vi "Main.vi"() -> ()   [LabVIEW 2016]
doc: "DACELL DN-10W load cell indicator \nmodbus communication program \n*function mode: Decision mode\n\nget display value\nget relay set value\nget physical unit\nset relay set value\n\nloop time 500 ms"
uses:
  Ctl/ctl_state.ctl
  <vilib>/NI/Modbus Library/API/Master/Modbus Master.lvclass
  <vilib>/Utility/error.llb/DialogType.ctl
panel:
  out "State":T1
  out "Error Out":errorcluster caption="에러 출력"
  in  "Error In":errorcluster caption="에러 입력"
  out "Run?":bool
  out "Connected?":bool
  in  "end":bool
  in  "zero":bool
  in  "update":bool
  in  "read":bool
  in  "disconnect":bool
  in  "connect":bool
  in  "Set velue":dbl=18.9 format="%#.1g"
  out "Unit":string="kgf"
  out "High limit":dbl
  out "Low limit":dbl
  out "relay3":bool
  out "relay2":bool
  out "relay1":bool
  out "Present value":dbl
  in  "baud rate":u32=9600
  in  "unit ID":u8=2
  in  "VISA resource name":refnum<visa-resource-name>
  # "DACELL DN-10W \nMODBUS Communication Program"
  # "DACELL DN-10W indicator MODBUS-RTU by Kyuman Kim"
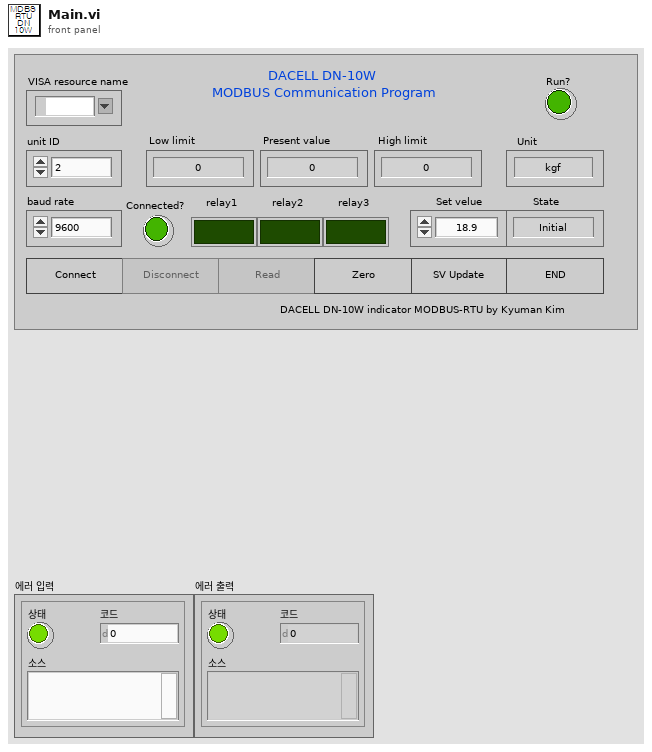
[diagram p1: front panel]
types:
  T1 = typedef "ctl_state.ctl" = enum16{"Initial", "Wait", "Connect", "Disconnect", "Read", "Update", "Zero", "End"}
  T2 = enum8{"Enabled", "Disabled", "Disabled and Grayed Out"}
  T3 = typedef "DialogType.ctl" = u16
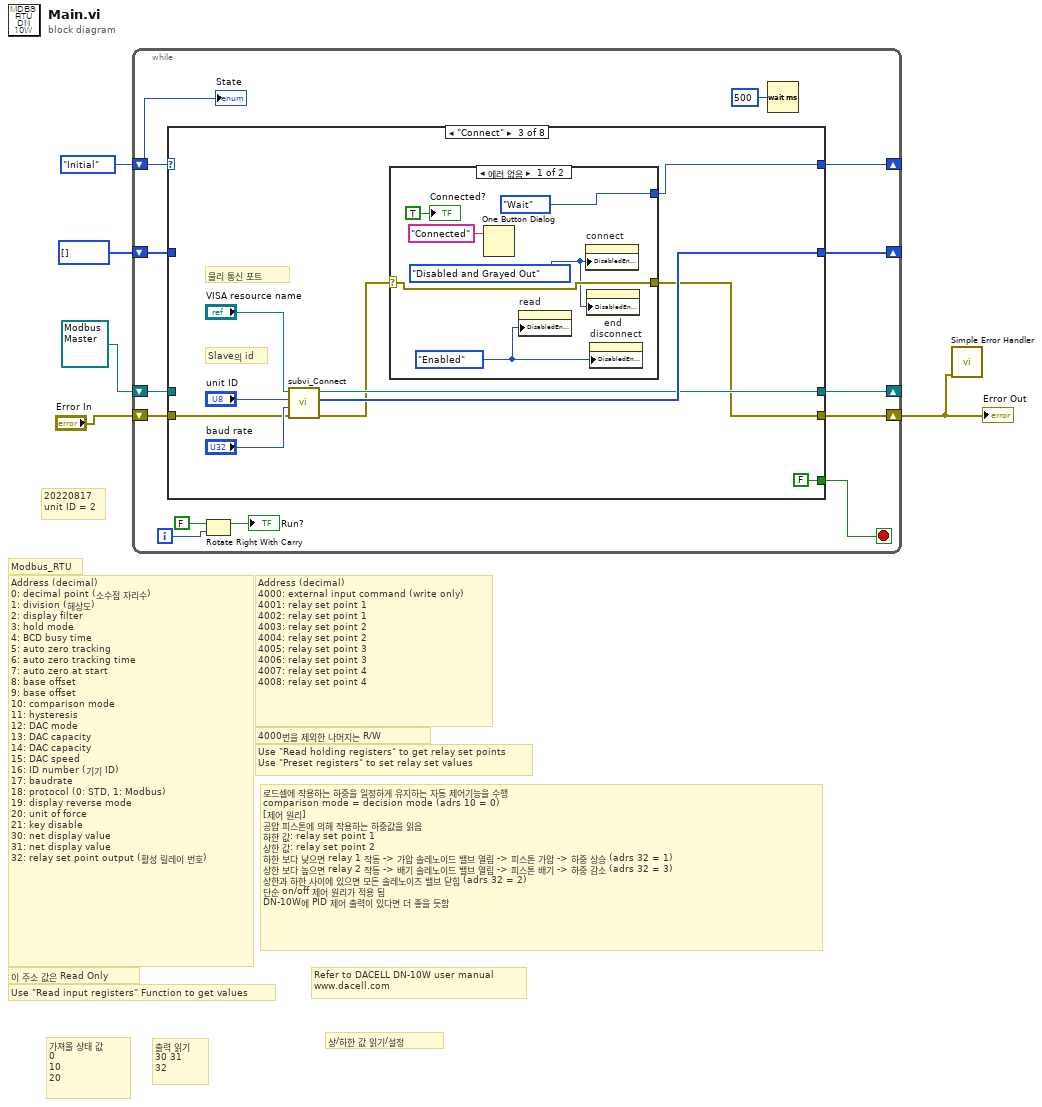
[diagram p0: block diagram]
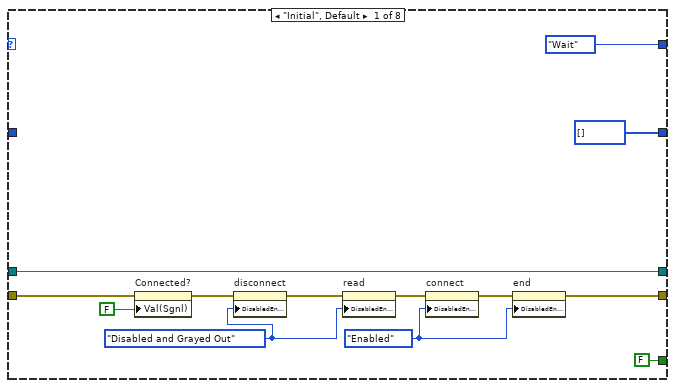
[diagram p2: hidden frame]
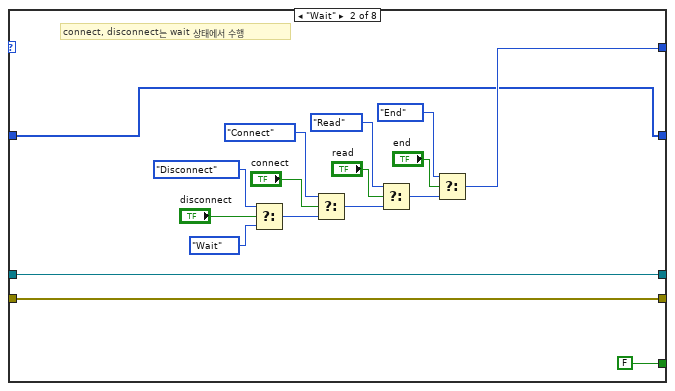
[diagram p3: hidden frame]
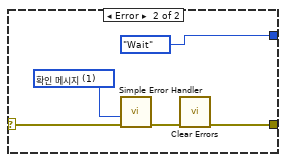
[diagram p4: hidden frame]
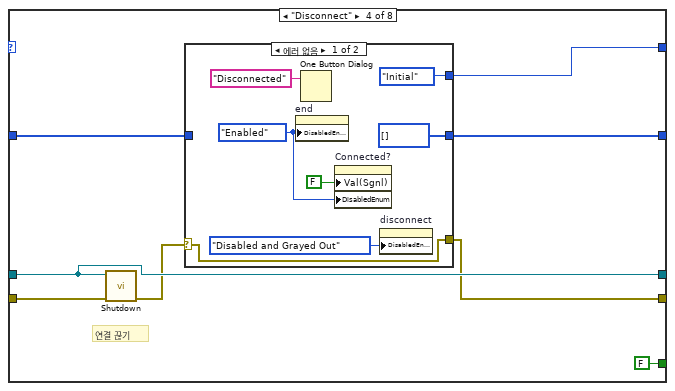
[diagram p5: hidden frame]
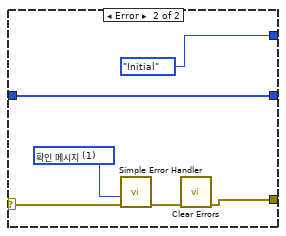
[diagram p6: hidden frame]
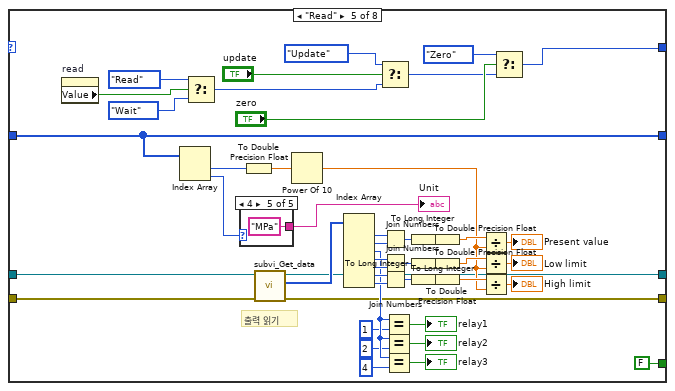
[diagram p7: hidden frame]
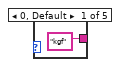
[diagram p8: hidden frame]
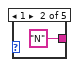
[diagram p9: hidden frame]
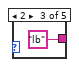
[diagram p10: hidden frame]
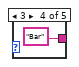
[diagram p11: hidden frame]
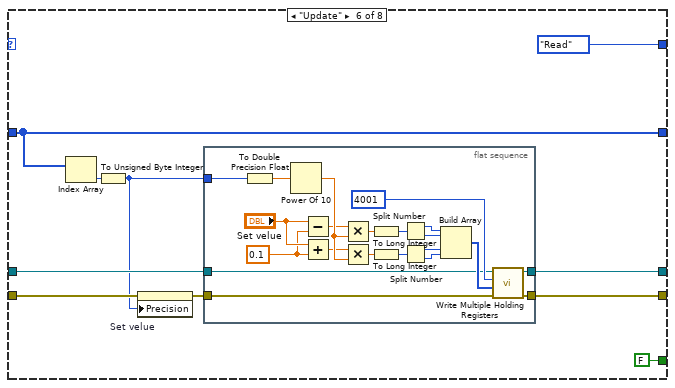
[diagram p12: hidden frame]
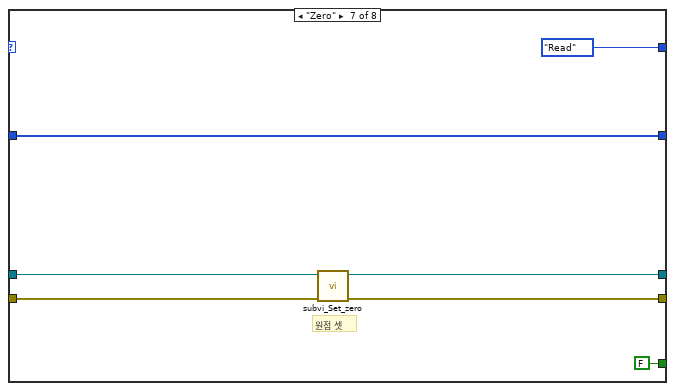
[diagram p13: hidden frame]
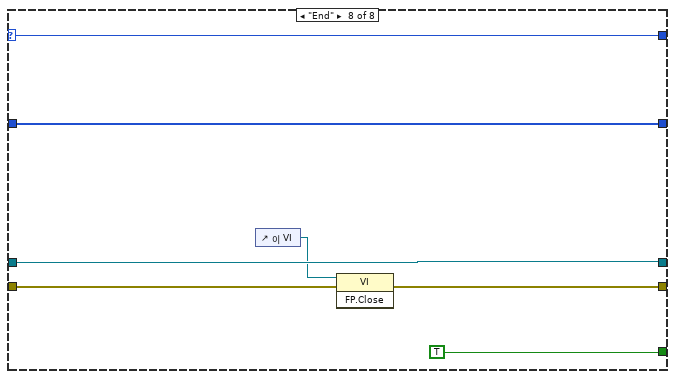
[diagram p14: hidden frame]
diagram:
  # "20220817\nunit ID = 2"
  # "상/하한 값 읽기/설정"
  # "출력 읽기\n30 31\n32"
  # "가져올 상태 값\n0\n10\n20"
  # "로드셀에 작용하는 하중을 일정하게 유지하는 자동 제어기능을 수행\ncomparison mode = decision mode (adrs 10 = 0)\n[제어 원리]\n공압 피스톤에 의해 작용하는 하중값을 읽음\n하한 값: relay set point 1\n상한 값: relay set point 2\n하한 보다 낮으면 relay 1 작동 -> 가압 솔레노이드 밸브 열림 -> 피스톤 가압 -> 하중 상승 (adrs 32 = 1)\n상한 보다 높으면 relay 2 작동 -> 배기 솔레노이드 밸브 열림 -> 피스톤 배기 -> 하중 감소 (adrs 32 = 3)\n상한과 하한 사이에 있으면 모든 솔레노이즈 밸브 닫힘 (adrs 32 = 2)\n단순 on/off 제어 원리가 적용 됨\nDN-10W에 PID 제어 출력이 있다면 더 좋을 듯함"
  # "4000번을 제외한 나머지는 R/W"
  # "이 주소 값은 Read Only"
  # "Modbus_RTU"
  # "Refer to DACELL DN-10W user manual\nwww.dacell.com"
  # "Use \"Read holding registers\" to get relay set points\nUse \"Preset registers\" to set relay set values"
  # "Use \"Read input registers\" Function to get values"
  # "Address (decimal)\n4000: external input command (write only)\n4001: relay set point 1 \n4002: relay set point 1\n4003: relay set point 2\n4004: relay set point 2\n4005: relay set point 3\n4006: relay set point 3\n4007: relay set point 4\n4008: relay set point 4"
  # "Address (decimal)\n0: decimal point (소수점 자리수)\n1: division (해상도)\n2: display filter\n3: hold mode\n4: BCD busy time\n5: auto zero tracking\n6: auto zero tracking time\n7: auto zero at start\n8: base offset\n9: base offset\n10: comparison mode \n11: hysteresis\n12: DAC mode\n13: DAC capacity\n14: DAC capacity\n15: DAC speed\n16: ID number (기기 ID)\n17: baudrate \n18: protocol (0: STD, 1: Modbus)\n19: display reverse mode\n20: unit of force\n21: key disable\n30: net display value \n31: net display value\n32: relay set point output (활성 릴레이 번호)"
  n1 = while {
    shift-right: [w16] -> w1
    shift-left: "Error In" -> [w17]
    shift-right: [w15] -> _
    shift-left: u16[] [] ("register values") -> [w12]
    shift-right: [w14] -> _
    shift-left: refnum<class "Modbus Master.lvclass"> refnum ("Modbus Master 출력") -> [w13]
    shift-right: [w11] -> _
    shift-left: ctl_state."Initial" ("열거형") -> [w18]
    i -> [w8]
    stop <- w10 stop-if-true
    n2 = case shown="\"Connect\"" w18 {
      selector: w18 -> [_ _ _ _ _ _ _ w184]
      tunnel: w17 -> [w23 w47 w55 w77 w91 w148 w178 w186]
      tunnel: [w19 w47 w49 w70 w106 w143 w174 w185] -> w16
      tunnel: [u16[] [] ("register values") w33 w54 w73 w103 w149 w177 w187] -> w15
      tunnel: [w31 w48 w53 w76 w104 w150 w179 w182] -> w14
      tunnel: w13 -> [w31 w48 _ w76 w105 w151 w180 w182]
      tunnel: w12 -> [_ w33 _ w74 w103 w149 w177 w187]
      tunnel: [ctl_state."Wait" ("열거형") w34 w52 w75 w94 ctl_state."Read" ("열거형") ctl_state."Read" ("열거형") w184] -> w11
      tunnel: [FALSE FALSE FALSE FALSE FALSE FALSE FALSE TRUE] -> w10
      frame "Initial", Default {
        w25 = T2."Enabled" ("비활성화")
        w26 = T2."Disabled and Grayed Out" ("비활성화")
        n3 = property on="Connected?" class="Bool (엄격한)"(error in=w23, "Val(Sgnl)"=FALSE ("값(신호)")) -> (error out=w30:errorcluster)  [unwired: 1 in, 1 out]
        n4 = property on="disconnect" class="Bool"(error in=w30, "DisabledEnum"=w26) -> (error out=w22:errorcluster)  [unwired: 1 in, 1 out]
        n5 = property on="read" class="Bool (엄격한)"(error in=w22, "DisabledEnum"=w26) -> (error out=w21:errorcluster)  [unwired: 1 in, 1 out]
        n6 = property on="connect" class="Bool"(error in=w21, "DisabledEnum"=w25) -> (error out=w20:errorcluster)  [unwired: 1 in, 1 out]
        n7 = property on="end" class="Bool"(error in=w20, "DisabledEnum"=w25) -> (error out=w19:errorcluster)  [unwired: 1 in, 1 out]
      }
      frame "Wait" {
        # "connect, disconnect는 wait 상태에서 수행"
        n8 = Select(t=ctl_state."Disconnect" ("열거형"), s="disconnect", f=ctl_state."Wait" ("열거형")) -> (s? t:f=w44:T1)
        n9 = Select(t=ctl_state."Connect" ("열거형"), s="connect", f=w44) -> (s? t:f=w40:T1)
        n10 = Select(t=ctl_state."Read" ("열거형"), s="read", f=w40) -> (s? t:f=w36:T1)
        n11 = Select(t=ctl_state."End" ("열거형"), s="end", f=w36) -> (s? t:f=w34:T1)
      }
      frame "Connect" {
        # "물리 통신 포트"
        # "Slave의 id"
        n12 = call "subvi_Connect.vi"("에러"=w55, "baud rate"="baud rate", "unit ID"="unit ID", "VISA 참조 번호 입력"="VISA resource name") -> ("에러 출력"=w50:errorcluster, "register values"=w54:u16[], "Modbus Master 출력"=w53:refnum<class "Modbus Master.lvclass">)  [unwired: 5 in]
        n13 = case shown="에러 없음" w50 {
          selector: w50 -> [w64 w68]
          tunnel: [ctl_state."Wait" ("열거형") ctl_state."Wait" ("열거형")] -> w52
          tunnel: [w64 w65] -> w49
          frame No Error {
            w59 = T2."Enabled" ("비활성화")
            w60 = T2."Disabled and Grayed Out" ("비활성화")
            n14 = One Button Dialog(message="Connected" ("메시지")) -> ()  [unwired: 1 in, 1 out]
            n15 = property on="read" class="Bool (엄격한)"("DisabledEnum"=w59) -> ()  [unwired: 2 in, 2 out]
            n16 = property on="connect" class="Bool"("DisabledEnum"=w60) -> ()  [unwired: 2 in, 2 out]
            n17 = property on="end" class="Bool"("DisabledEnum"=w60) -> ()  [unwired: 2 in, 2 out]
            n18 = property on="disconnect" class="Bool"("DisabledEnum"=w59) -> ()  [unwired: 2 in, 2 out]
            "Connected?" <- TRUE ("Connected?")
          }
          frame Error {
            w67 = T3 1 items=["대화 상자 없음", "확인 메시지", "메시지 지속 또는 정지", "확인 메시지 + 경고", "지속/정지 + 경고"] ("type of dialog (OK msg:1)")
            n19 = call <vilib>:"Simple Error Handler.vi"("type of dialog (OK msg:1)"=w67, "error in (no error)"=w68) -> ("error out"=w66:errorcluster)  [unwired: 3 in, 4 out]
            n20 = call <vilib>:"Clear Errors.vi"("error in (no error)"=w66) -> ("error out"=w65:errorcluster)  [unwired: 5 in, 1 out]
          }
        }
      }
      frame "Disconnect" {
        # "연결 끊기"
        n21 = call-dynamic "Shutdown.vi"("error in"=w77, "Modbus master in"=w76) -> ("error out"=w71:errorcluster)  [unwired: 9 in]
        n22 = case shown="에러 없음" w71 {
          selector: w71 -> [w78 w89]
          tunnel: [ctl_state."Initial" ("열거형") ctl_state."Initial" ("열거형")] -> w75
          tunnel: w74 -> [_ w87]
          tunnel: [u16[] [] ("register values") w87] -> w73
          tunnel: [w78 w85] -> w70
          frame No Error {
            w80 = T2."Enabled" ("비활성화")
            n23 = property on="end" class="Bool"("DisabledEnum"=w80) -> ()  [unwired: 2 in, 2 out]
            n24 = One Button Dialog(message="Disconnected" ("메시지")) -> ()  [unwired: 1 in, 1 out]
            n25 = property on="Connected?" class="Bool (엄격한)"("Val(Sgnl)"=FALSE ("값(신호)"), "DisabledEnum"=w80) -> ()  [unwired: 2 in, 2 out]
            n26 = property on="disconnect" class="Bool"("DisabledEnum"=T2."Disabled and Grayed Out" ("비활성화")) -> ()  [unwired: 2 in, 2 out]
          }
          frame Error {
            w88 = T3 1 items=["대화 상자 없음", "확인 메시지", "메시지 지속 또는 정지", "확인 메시지 + 경고", "지속/정지 + 경고"] ("type of dialog (OK msg:1)")
            n27 = call <vilib>:"Simple Error Handler.vi"("type of dialog (OK msg:1)"=w88, "error in (no error)"=w89) -> ("error out"=w86:errorcluster)  [unwired: 3 in, 4 out]
            n28 = call <vilib>:"Clear Errors.vi"("error in (no error)"=w86) -> ("error out"=w85:errorcluster)  [unwired: 5 in, 1 out]
          }
        }
      }
      frame "Read" {
        # "출력 읽기"
        n29 = property on="read" class="Bool (엄격한)"() -> ("Value"=w93:bool)  [unwired: 2 in, 2 out]
        n30 = Index Array(array=w103) -> (element #1=w137:u16, element #2=w125:u16)  [unwired: 2 in]
        n31 = Select(t=ctl_state."Read" ("열거형"), s=w93, f=ctl_state."Wait" ("열거형")) -> (s? t:f=w98:T1)
        n32 = case shown="4" w125 {
          tunnel: ["kgf" "N" "lb" "Bar" "MPa"] -> w124
          frame 0, Default {
          }
          frame 1 {
          }
          frame 2 {
          }
          frame 3 {
          }
          frame 4 {
          }
        }
        "Unit" <- w124
        n33 = To Double Precision Float(number=w137) -> (double precision float=w123:dbl)
        n34 = call "subvi_Get_data.vi"("에러 입력(에러 없음)"=w91, "Modbus Master 입력"=w105) -> ("에러 출력"=w106:errorcluster, "register values"=w107:u16[], "Modbus Master 출력"=w104:refnum<class "Modbus Master.lvclass">)  [unwired: 7 in]
        n35 = Power Of 10(x=w123) -> (10^x=w133:dbl)
        n36 = Index Array(array=w107) -> (element #1=w109:u16, element #2=w108:u16, element #3=w115:u16, element #4=w126:u16, element #5=w127:u16, element #6=w128:u16, element #7=w129:u16)  [unwired: 7 in]
        n37 = Select(t=ctl_state."Update" ("열거형"), s="update", f=w98) -> (s? t:f=w95:T1)
        n38 = Join Numbers(hi=w109, lo=w108) -> ((hi.lo)=w110:u32)
        n39 = Join Numbers(hi=w126, lo=w127) -> ((hi.lo)=w119:u32)
        n40 = Join Numbers(hi=w128, lo=w129) -> ((hi.lo)=w120:u32)
        n41 = Equal?(x=w115, y=u16 1) -> (x = y?=→"relay1":bool)
        n42 = Equal?(x=w115, y=u16 2) -> (x = y?=→"relay2":bool)
        n43 = Equal?(x=w115, y=u16 4) -> (x = y?=→"relay3":bool)
        n44 = To Long Integer(number=w110) -> (32bit integer=w111:i32)
        n45 = To Long Integer(number=w119) -> (32bit integer=w121:i32)
        n46 = To Long Integer(number=w120) -> (32bit integer=w122:i32)
        n47 = To Double Precision Float(number=w111) -> (double precision float=w134:dbl)
        n48 = To Double Precision Float(number=w121) -> (double precision float=w135:dbl)
        n49 = To Double Precision Float(number=w122) -> (double precision float=w136:dbl)
        n50 = Divide(x=w134, y=w133) -> (x/y=→"Present value":dbl)
        n51 = Divide(x=w135, y=w133) -> (x/y=→"Low limit":dbl)
        n52 = Divide(x=w136, y=w133) -> (x/y=→"High limit":dbl)
        n53 = Select(t=ctl_state."Zero" ("열거형"), s="zero", f=w95) -> (s? t:f=w94:T1)
      }
      frame "Update" {
        n54 = Index Array(array=w149) -> (element=w152:u16)  [unwired: 1 in]
        n55 = To Unsigned Byte Integer(number=w152) -> (unsigned 8bit integer=w146:u8)
        n56 = property on="Set velue" class="DigNum (엄격한)"(error in=w148, "Precision"=w146) -> (error out=w147:errorcluster)  [unwired: 1 in, 1 out]
        n57 = flat-sequence {
          tunnel: w151 -> [w161]
          tunnel: [w160] -> w150
          tunnel: [w159] -> w143
          tunnel: w147 -> [w154]
          tunnel: w146 -> [w153]
          frame #0 {
            w157 = 0.1
            n58 = To Double Precision Float(number=w153) -> (double precision float=w164:dbl)
            n59 = Power Of 10(x=w164) -> (10^x=w168:dbl)
            n60 = Subtract(x="Set velue", y=w157) -> (x-y=w155:dbl)
            n61 = Add(x="Set velue", y=w157) -> (x+y=w156:dbl)
            n62 = Multiply(x=w155, y=w168) -> (x*y=w167:dbl)
            n63 = Multiply(x=w156, y=w168) -> (x*y=w166:dbl)
            n64 = To Long Integer(number=w167) -> (32bit integer=w163:i32)
            n65 = To Long Integer(number=w166) -> (32bit integer=w165:i32)
            n66 = Split Number(x=w163) -> (hi(x)=w169:u16, lo(x)=w170:u16)
            n67 = Split Number(x=w165) -> (hi(x)=w171:u16, lo(x)=w172:u16)
            n68 = Build Array(w169, w170, w171, w172) -> (w173:u16[])
            n69 = call-dynamic "Write Multiple Holding Registers.vi"("error in"=w154, "registers to write"=w173, "starting address"=u16 4001, "Modbus master in"=w161) -> ("error out"=w159:errorcluster, "Modbus master out"=w160:refnum<class "Modbus Master.lvclass">)  [unwired: 6 in]
          }
        }
      }
      frame "Zero" {
        # "원점 셋"
        n70 = call "subvi_Set_zero.vi"("에러 입력(에러 없음)"=w178, "Modbus Master 입력"=w180) -> ("에러 출력"=w174:errorcluster, "Modbus Master 출력"=w179:refnum<class "Modbus Master.lvclass">)  [unwired: 8 in]
      }
      frame "End" {
        n71 = control-ref of="이 VI"() -> (w181:refnum<vi>)
        n72 = invoke class="VI" method="FP.Close"(reference=w181, error in=w186) -> (error out=w185:errorcluster)  [unwired: 1 in, 2 out]
      }
    }
    n73 = Rotate Right With Carry(2:w8, 3:FALSE ("캐리")) -> (1:→"Run?":bool)  [unwired: 1 out]
    n74 = Wait (ms)(milliseconds to wait=u32 500 ("대기 시간 (ms)")) -> ()  [unwired: 1 out]
    "State" <- w18
  }
  "Error Out" <- w1
  n75 = call <vilib>:"Simple Error Handler.vi"("error in (no error)"=w1) -> ()  [unwired: 4 in, 5 out]
